vi "Laser Parameters.vi"() -> ()   [LabVIEW 2020]
panel:
  in  "REST port":string="35100"
  in  "Laser IP":string="10.0.40.83"
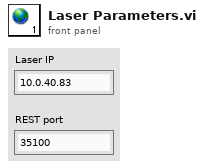
[diagram p1: front panel]
diagram:
